vi "lick-read-debug.vi"() -> (2 "Lick Status":bool)   [LabVIEW 2015]
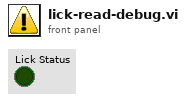
[diagram p1: front panel]
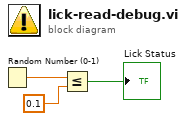
[diagram p0: block diagram]
diagram:
  n1 = Random Number (0-1)() -> (number: 0 to 1=w3:dbl)
  n2 = Less Or Equal?(x=w3, y=0.1) -> (x <= y?=→"Lick Status":bool)
